vi "Read Integer.vi"(7 "Section":string, 8 "error in":errorcluster, 10 "Key":string, 11 "config-base in":refnum<class "config-base.lvclass">) -> (0 "error out":errorcluster, 2 "Value":i64, 3 "config-base out":refnum<class "config-base.lvclass">)   [LabVIEW 2020, in "hse-config.lvlib" / "config-base.lvclass"]
doc: "Returns a integer (I64) config key.\n\n____\nHAMPEL SOFTWARE ENGINEERING v3.8.0 (2023-12-18 14:41)"
uses:
  config-base.lvclass
  <vilib>/Utility/Data Type/Type Definitions/Data Type.ctl
  config-base.lvclass/config-base.ctl
  <vilib>/Utility/Data Type/NI_Data Type.lvlib
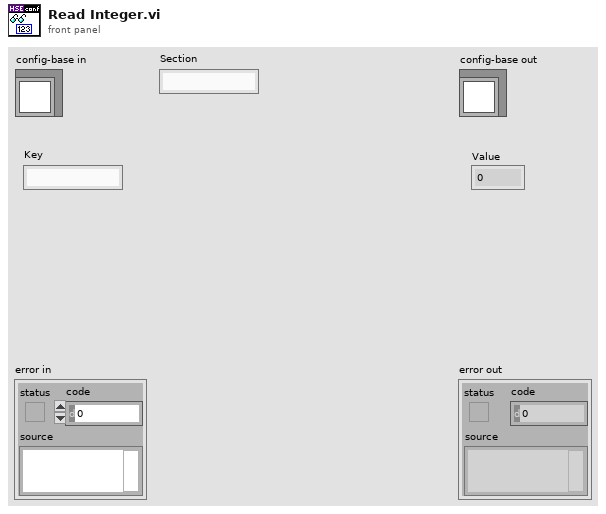
[diagram p1: front panel]
types:
  T1 = typedef "NI_Data Type.lvlib/Data Type.ctl" = enum8{"Invalid Type", "Void", "I8", "I16", "I32", "I64", "U8", "U16", "U32", "U64", "Single Float", "Double Float", "Extended Float", "Single Complex", "Double Complex", "Extended Complex", "Enum U8", "Enum U16", "Enum U32", "Enum U64", "Single Float With Unit", "Double Float With Unit", "Extended Float With Unit", "Single Complex with Unit", "Double Complex with Unit", "Extended Complex with Unit", "Boolean", "String", "Path", "Picture", "Tag", "Array", "Cluster", "Variant", "LV Variant", "Waveform", "Timestamp", "Digital Waveform", "Digital Data", "ExpressData", "Refnum", "External Data", "VI", "Poly VI", "LabVIEW Class Instance", "Fixed Point", "Set Collection", "Map Collection"}
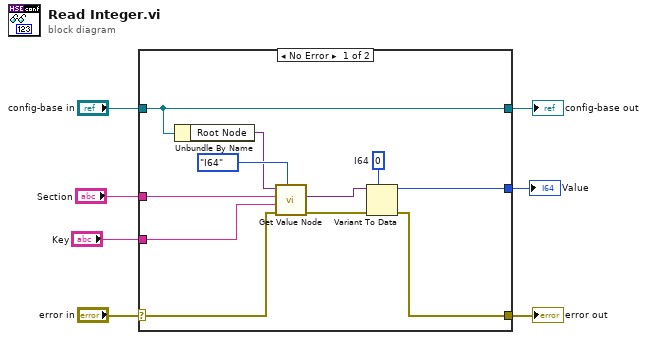
[diagram p0: block diagram]
diagram:
  n1 = case shown="No Error" "error in" {
    selector: "error in" -> [w11 w20]
    tunnel: [w10 w20] -> w6
    tunnel: [w15 w19] -> w4
    tunnel: "config-base in" -> [w15 w19]
    tunnel: "Section" -> [w13 _]
    tunnel: "Key" -> [w12 _]
    tunnel: [w8 _] -> w1
    frame No Error {
      w9 = i64 0  # I64
      n2 = Unbundle By Name(w15) -> ("Root Node"=w14:variant)
      n3 = call "Get Value Node.vi"("Data Type"=Data_Type."I64", "error in"=w11, "Key"=w12, "Section"=w13, "Root Node"=w14) -> ("error out"=w17:errorcluster, "Value Node out"=w18:variant)  [unwired: 5 in]
      n4 = Variant To Data(error in=w17, type=w9, Variant=w18) -> (data=w8:i64, error out=w10:errorcluster)
    }
    frame Error {
    }
  }
  "error out" <- w6
  "config-base out" <- w4
  "Value" <- w1
